vi "Read Model from JSON.vi"(8 "error in (no error)":errorcluster, 11 "JSON string":string) -> (0 "error out":errorcluster, 1 "threshold for anomaly detection":T1, 3 "model out":refnum<class "AML Analytics Model.lvclass">, 4 "custom info":cluster{"key":string, "value":string}[](array[cluster]))   [LabVIEW 2017, in "MachineLearning.lvlib"]
doc: "Converts the JSON string from a saved model file to a model reference for deployment."
uses:
  MachineLearning.lvlib
  <vilib>/addons/AML/Common/Classes/AML Analytics Model.lvclass
  <vilib>/addons/AML/Example Support/aml_All Models (enum).ctl
  <vilib>/addons/AML/Feature Manipulation/Common/Controls/aml_Feature Manipulation Model Type.ctl
  <vilib>/addons/AML/Anomaly Detection/Common/Controls/aml_Anomaly Detection Model Type.ctl
  <vilib>/addons/AML/Clustering/Common/Controls/aml_Clustering Model Type.ctl
  <vilib>/addons/AML/Classification/Common/Controls/aml_Classification Model Type.ctl
  TypeDefs/JSONpath.ctl
  TypeDefs/All Models.ctl
  <vilib>/addons/AML/Feature Manipulation/PCA/Controls/aml_PCA Properties.ctl
  <vilib>/addons/AML/Anomaly Detection/PCA T2Q/Controls/aml_PCA T2Q Properties.ctl
  <vilib>/addons/AML/Anomaly Detection/GMM-CV/Controls/aml_ GMM-CV Model Parameters.ctl
  <vilib>/addons/AML/Clustering/GMM/Controls/aml_GMM Parameter.ctl
  <vilib>/addons/AML/Anomaly Detection/GMM-CV/Controls/aml_ GMM-CV Trained Model.ctl
  <vilib>/addons/AML/Clustering/DBSCAN/Controls/aml_DBSCAN Model.ctl
  <vilib>/addons/AML/Clustering/K-Means/Controls/aml_Kmeans Model.ctl
  <vilib>/addons/AML/Clustering/GMM/Controls/aml_GMM Model.ctl
  <vilib>/addons/AML/Classification/Logistic Regression/Controls/aml_Logistic Regression Model.ctl
  <vilib>/addons/AML/Classification/Common/Classes/AML Classification.lvclass/AML Classification.ctl
  <vilib>/addons/AML/Classification/Logistic Regression/Classes/AML Logistic Regression.lvclass/AML Logistic Regression.ctl
  <vilib>/addons/AML/Common/Classes/AML Analytics Model.lvclass/AML Analytics Model.ctl
  <vilib>/addons/AML/Classification/Set Classification Model (LR).vi
  <vilib>/addons/AML/Classification/Logistic Regression/Classes/aml_Write Coefficients.vi
  <vilib>/addons/AML/Classification/Common/Classes/aml_Write Number of Classes.vi
  <vilib>/addons/AML/Classification/Common/Classes/aml_Write Label of Each Class.vi
  <vilib>/addons/AML/Common/Classes/aml_Write AML Classification Model.vi
  <vilib>/addons/AML/Classification/Common/Classes/aml_Write Model Status.vi
  <vilib>/addons/AML/Classification/Common/Classes/aml_Write Classification Model Type.vi
  <vilib>/addons/AML/Common/Classes/aml_Write Classification Model Type.vi
  <vilib>/addons/AML/Classification/Common/Classes/aml_Read Classification Model Type.vi
  <vilib>/addons/AML/Classification/Logistic Regression/Classes/AML Logistic Regression.lvclass
  C:/Program Files (x86)/National Instruments/LabVIEW 2017/vi.lib/addons/AML/Classification/Common/Classes/AML Classification.lvclass
  <vilib>/addons/AML/Classification/Logistic Regression/subVIs/aml_Check LR Model.vi
  <vilib>/addons/AML/Classification/Set Classification Model (NN).vi
  <vilib>/addons/AML/Classification/Set Classification Model (SVM).vi
  <vilib>/addons/AML/Clustering/Set Clustering Model (GMM).vi
  <vilib>/addons/AML/Clustering/Set Clustering Model (K-Means).vi
  <vilib>/addons/AML/Clustering/Set Clustering Model (DBSCAN).vi
  <vilib>/addons/AML/Anomaly Detection/Set Anomaly Detection Model (One-Class SVM).vi
  <vilib>/addons/AML/Anomaly Detection/Set Anomaly Detection Model (GMM-CV).vi
  <vilib>/addons/AML/Anomaly Detection/Set Anomaly Detection Model (PCA T2Q).vi
  <vilib>/addons/AML/Anomaly Detection/Set Anomaly Detection Model (SOM-MQE).vi
  <vilib>/addons/AML/Feature Manipulation/Set Feature Manipulation Model (KPCA).vi
  <vilib>/addons/AML/Feature Manipulation/Set Feature Manipulation Model (PCA).vi
  <vilib>/addons/AML/Feature Manipulation/Set Feature Manipulation Model (Fisher).vi
  <vilib>/addons/AML/Feature Manipulation/Set Feature Manipulation Model (Normalize).vi
  <vilib>/addons/AML/Analytics and Machine Learning.lvlib
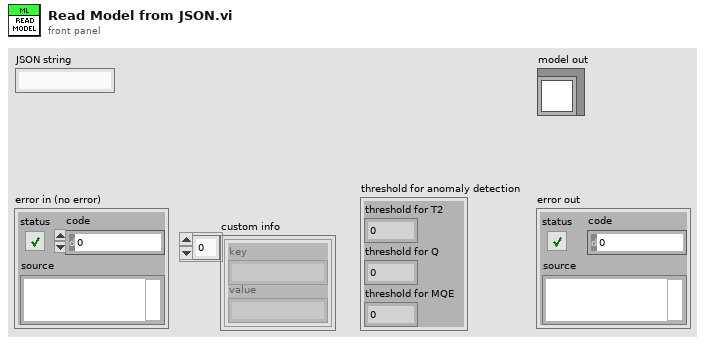
[diagram p1: front panel]
types:
  T1 = cluster{"threshold for T2":dbl, "threshold for Q":dbl, "threshold for MQE":dbl}
  T2 = typedef "All Models.ctl" = cluster{u16[], u16, u16, u16}
  T3 = typedef "MachineLearning.lvlib/JSONpath.ctl" = enum16{"Training Time", "All Models", "Feature Manipulation", "Anomaly Detection", "Clustering", "Classification", "Custom Info"}
  T4 = typedef "aml_All Models (enum).ctl" = cluster{"feature manipulation":T5[], "anomaly detection model type":T6, "clustering model type":T7, "classification model type":T8}
  T5 = typedef "Analytics and Machine Learning.lvlib/aml_Feature Manipulation Model Type.ctl" = enum16{"None", "Normalize", "Fisher", "PCA", "KPCA"}
  T6 = typedef "Analytics and Machine Learning.lvlib/aml_Anomaly Detection Model Type.ctl" = enum16{"None", "SOM-MQE", "PCA T2Q", "GMM-CV", "One-class SVM"}
  T7 = typedef "Analytics and Machine Learning.lvlib/aml_Clustering Model Type.ctl" = enum16{"None", "DBSCAN", "K-Means", "GMM"}
  T8 = typedef "Analytics and Machine Learning.lvlib/aml_Classification Model Type.ctl" = enum16{"None", "SVM", "Neural Network", "Logistic Regression", "Multi-Layer Neural Network"}
  T9 = cluster{"normalization settings":cluster{"transformation method":i32, "range settings":cluster{"max":dbl, "min":dbl}}, "mean values":dbl[], "standard deviation values":dbl[], "min values":dbl[], "max values":dbl[]}
  T10 = typedef "Analytics and Machine Learning.lvlib/aml_PCA Properties.ctl" = cluster{"mean values":dbl[], "eigenvectors":dbl[][]}
  T11 = cluster{"kernel settings":cluster{"type":i32, "degree":i32, "gamma":dbl, "coef0":dbl}, "variance":dbl[], "source data":dbl[][], "eigenvectors":dbl[][]}
  T12 = cluster{"map vectors":dbl[][], "MQE threshold":dbl, "map structure":cluster{"row":i32, "col":i32, "lattice type":i32}}
  T13 = typedef "Analytics and Machine Learning.lvlib/aml_PCA T2Q Properties.ctl" = cluster{"mean values":dbl[], "eigenvectors":dbl[][], "variance":dbl[], "threshold for T2":dbl, "threshold for Q":dbl}
  T14 = typedef "Analytics and Machine Learning.lvlib/aml_ GMM-CV Model Parameters.ctl" = cluster{"hyperparameters":T15, "baseline model":T16}
  T15 = typedef "Analytics and Machine Learning.lvlib/aml_GMM Parameter.ctl" = cluster{"auto initialization":bool, "initial mean values":dbl[][], "initial covariance values":cluster{"initial covariance matrix":dbl[][]}[], "initial weights":dbl[], "number of clusters":i32, "regulator":dbl, "tolerance":dbl, "max iteration":i32}
  T16 = typedef "Analytics and Machine Learning.lvlib/aml_ GMM-CV Trained Model.ctl" = cluster{"weights":dbl[], "covariance values":cluster{"covariance matrix":dbl[][]}[], "mean values":dbl[][]}
  T17 = cluster{"kernel settings":cluster{"type":i32, "degree":i32, "gamma":dbl, "coef0":dbl}, "number of support vectors":i32, "support vectors":dbl[][], "coeffcients of support vectors":dbl[][], "decision function constants":dbl[]}
  T18 = typedef "Analytics and Machine Learning.lvlib/aml_DBSCAN Model.ctl" = cluster{"max distance":dbl, "p":dbl, "core samples":dbl[][], "core samples labels":i32[]}
  T19 = typedef "Analytics and Machine Learning.lvlib/aml_Kmeans Model.ctl" = cluster{"centroids":dbl[][], "number of clusters":i32}
  T20 = typedef "Analytics and Machine Learning.lvlib/aml_GMM Model.ctl" = cluster{"number of clusters":i32, "mean values":dbl[][], "covariance values":cluster{"covariance matrix":dbl[][]}[], "weights":dbl[]}
  T21 = cluster{"kernel settings":cluster{"type":dbl, "degree":i32, "gamma":dbl, "coef0":dbl}, "number of classes":i32, "label of each class":i32[], "number of support vectors":i32, "support vectors":dbl[][], "coeffcients of support vectors":dbl[][], "decision function constants":dbl[], "pairwise probability":cluster{"probA":dbl[], "probB":dbl[]}, "number of support vectors for each class":i32[]}
  T22 = cluster{"number of classes":i32, "label of each class":i32[], "number of input neurons":i32, "number of hidden neurons":i32, "number of output neurons":i32, "hidden layer type":i32, "output layer type":i32, "I to H coefficients":dbl[][], "H to O coefficients":dbl[][]}
  T23 = typedef "Analytics and Machine Learning.lvlib/aml_Logistic Regression Model.ctl" = cluster{"number of classes":i32, "label of each class":i32[], "coefficients":dbl[][]}
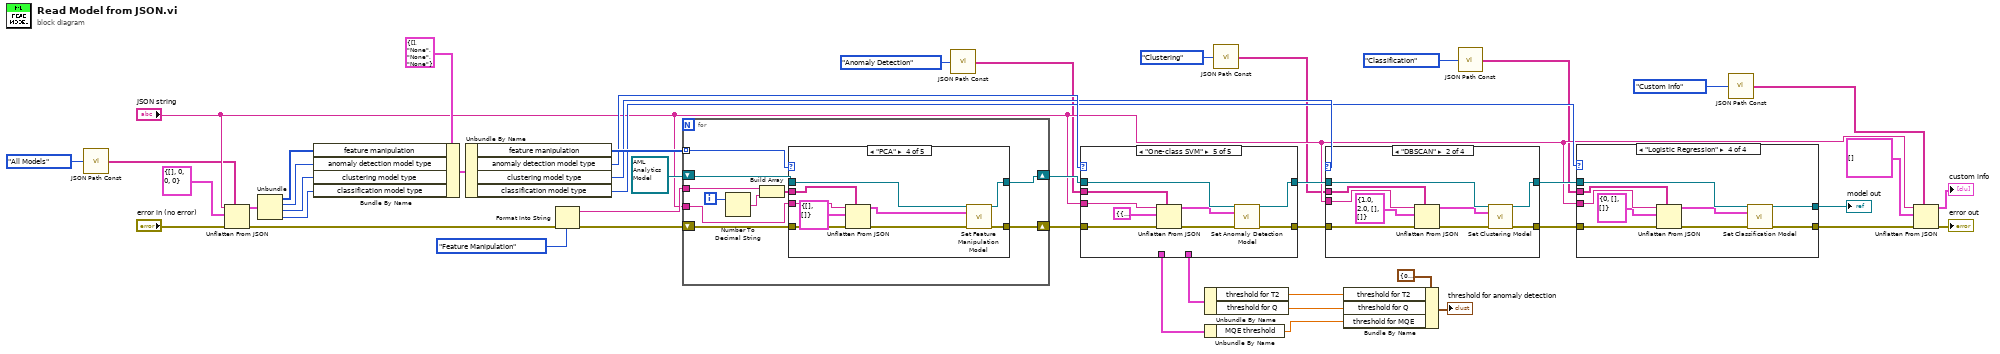
[diagram p0: block diagram]
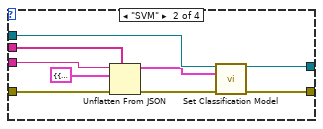
[diagram p3: hidden frame]
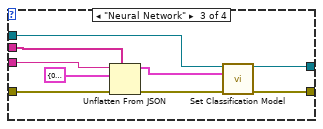
[diagram p4: hidden frame]
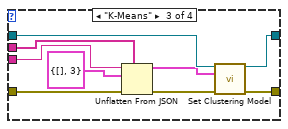
[diagram p6: hidden frame]
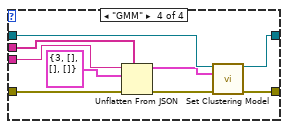
[diagram p7: hidden frame]
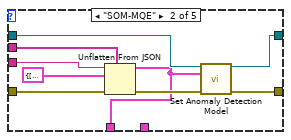
[diagram p9: hidden frame]
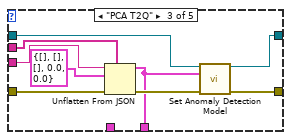
[diagram p10: hidden frame]
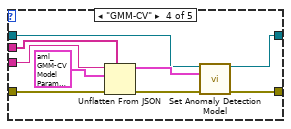
[diagram p11: hidden frame]
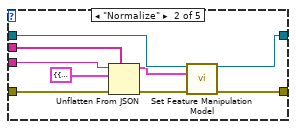
[diagram p13: hidden frame]
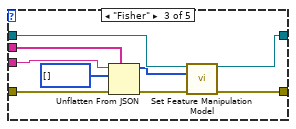
[diagram p14: hidden frame]
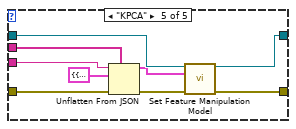
[diagram p15: hidden frame]
diagram:
  n1 = call "JSON Path Const.vi"("JSON Path"=JSONpath."All Models") -> ("resulting array"=w11:string[])
  n2 = Unflatten From JSON(path=w11, JSON string="JSON string", type and defaults=T2 {[], 0, 0, 0} ("cluster"), error in (no error)="error in (no error)") -> (value=w46:T2, error out=w26:errorcluster)  [unwired: 3 in]
  n3 = Unbundle(w46) -> (w41:u16[], w44:u16, w43:u16, w42:u16)
  n4 = Bundle By Name(cluster=T4 {"feature manipulation"=[], "anomaly detection model type"=enum."None", "clustering model type"=enum."None", "classification model type"=enum."None"}, "feature manipulation"=w41, "anomaly detection model type"=w44, "clustering model type"=w43, "classification model type"=w42) -> (w39:T4)
  n5 = Unbundle By Name(w39) -> ("feature manipulation"=w38:T5[], "anomaly detection model type"=w37:T6, "clustering model type"=w34:T7, "classification model type"=w30:T8)
  n6 = Format Into String(JSONpath."Feature Manipulation" ("JSON Path")) -> (resulting string=w28:string)  [unwired: 3 in, 1 out]
  n7 = for {
    tunnel: w38 -> [w47] mode=indexing
    tunnel: "JSON string" -> [w56]
    shift-right: [w54] -> w35
    shift-left: refnum<class "AML Analytics Model.lvclass"> refnum ("model out") -> [w55]
    shift-right: [w53] -> w36
    shift-left: w26 -> [w48]
    tunnel: w28 -> [w50]
    i -> [w52]
    n8 = Number To Decimal String(number=w52) -> (decimal integer string=w51:string)  [unwired: 1 in]
    n9 = Build Array(w50, w51) -> (w49:string[])
    n10 = case shown="\"PCA\"" w47 {
      tunnel: w56 -> [_ w67 w76 w85 w94]
      tunnel: w55 -> [w58 w66 w75 w84 w93]
      tunnel: [w58 w65 w74 w83 w92] -> w54
      tunnel: [w57 w63 w72 w81 w90] -> w53
      tunnel: w49 -> [_ w62 w71 w80 w89]
      tunnel: w48 -> [w57 w61 w70 w79 w88]
      frame "None", Default {
      }
      frame "Normalize" {
        n11 = Unflatten From JSON(path=w62, JSON string=w67, type and defaults=T9 {"normalization settings"={"transformation method"=0, "range settings"={"max"=0.0, "min"=0.0}}, "mean values"=[], "standard deviation values"=[], "min values"=[], "max values"=[]} ("normalization properties"), error in (no error)=w61) -> (value=w60:T9, error out=w64:errorcluster)  [unwired: 3 in]
        n12 = call-poly <vilib>:"Set Feature Manipulation Model.vi"("model in"=w66, "normalization model"=w60, "error in (no error)"=w64) -> ("model out"=w65:refnum<class "AML Analytics Model.lvclass">, "error out"=w63:errorcluster)  [unwired: 11 in]
      }
      frame "Fisher" {
        n13 = Unflatten From JSON(path=w71, JSON string=w76, type and defaults=i32[] [] ("Selected Feature Index"), error in (no error)=w70) -> (value=w68:i32[], error out=w73:errorcluster)  [unwired: 3 in]
        n14 = call-poly <vilib>:"Set Feature Manipulation Model.vi"("model in"=w75, "selected feature index"=w68, "error in (no error)"=w73) -> ("model out"=w74:refnum<class "AML Analytics Model.lvclass">, "error out"=w72:errorcluster)  [unwired: 11 in]
      }
      frame "PCA" {
        n15 = Unflatten From JSON(path=w80, JSON string=w85, type and defaults=T10 {"mean values"=[], "eigenvectors"=[]} ("PCA properties"), error in (no error)=w79) -> (value=w77:T10, error out=w82:errorcluster)  [unwired: 3 in]
        n16 = call-poly <vilib>:"Set Feature Manipulation Model.vi"("model in"=w84, "PCA model"=w77, "error in (no error)"=w82) -> ("model out"=w83:refnum<class "AML Analytics Model.lvclass">, "error out"=w81:errorcluster)  [unwired: 11 in]
      }
      frame "KPCA" {
        n17 = Unflatten From JSON(path=w89, JSON string=w94, type and defaults=T11 {"kernel settings"={"type"=0, "degree"=3, "gamma"=1.0, "coef0"=0.0}, "variance"=[], "source data"=[], "eigenvectors"=[]} ("KPCA properties"), error in (no error)=w88) -> (value=w86:T11, error out=w91:errorcluster)  [unwired: 3 in]
        n18 = call-poly <vilib>:"Set Feature Manipulation Model.vi"("model in"=w93, "KPCA model"=w86, "error in (no error)"=w91) -> ("model out"=w92:refnum<class "AML Analytics Model.lvclass">, "error out"=w90:errorcluster)  [unwired: 11 in]
      }
    }
  }
  n19 = call "JSON Path Const.vi"("JSON Path"=JSONpath."Anomaly Detection") -> ("resulting array"=w9:string[])
  n20 = case shown="\"One-class SVM\"" w37 {
    tunnel: w36 -> [w95 w105 w114 w123 w132]
    tunnel: w35 -> [w96 w104 w113 w121 w131]
    tunnel: [w96 w103 w112 w120 w130] -> w33
    tunnel: [w95 w101 w110 w118 w128] -> w32
    tunnel: "JSON string" -> [_ w100 w109 w117 w127]
    tunnel: w9 -> [_ w99 w108 w116 w126]
    tunnel: [_ _ w106 _ _] -> w19
    tunnel: [_ w97 _ _ _] -> w18
    frame "None", Default {
    }
    frame "SOM-MQE" {
      n21 = Unflatten From JSON(path=w99, JSON string=w100, type and defaults=T12 {"map vectors"=[], "MQE threshold"=0.0, "map structure"={"row"=0, "col"=0, "lattice type"=0}} ("SOM-MQE model"), error in (no error)=w105) -> (value=w97:T12, error out=w102:errorcluster)  [unwired: 3 in]
      n22 = call-poly <vilib>:"Set Anomaly Detection Model.vi"("model in"=w104, "SOM baseline model"=w97, "error in (no error)"=w102) -> ("model out"=w103:refnum<class "AML Analytics Model.lvclass">, "error out"=w101:errorcluster)  [unwired: 11 in]
    }
    frame "PCA T2Q" {
      n23 = Unflatten From JSON(path=w108, JSON string=w109, type and defaults=T13 {"mean values"=[], "eigenvectors"=[], "variance"=[], "threshold for T2"=0.0, "threshold for Q"=0.0} ("PCA T2Q model"), error in (no error)=w114) -> (value=w106:T13, error out=w111:errorcluster)  [unwired: 3 in]
      n24 = call-poly <vilib>:"Set Anomaly Detection Model.vi"("model in"=w113, "PCA baseline model"=w106, "error in (no error)"=w111) -> ("model out"=w112:refnum<class "AML Analytics Model.lvclass">, "error out"=w110:errorcluster)  [unwired: 11 in]
    }
    frame "GMM-CV" {
      n25 = Unflatten From JSON(path=w116, JSON string=w117, type and defaults=T14 {"hyperparameters"={"auto initialization"=TRUE, "initial mean values"=[], "initial covariance values"=[], "initial weights"=[], "number of clusters"=3, "regulator"=1e-06, "tolerance"=1e-05, "max iteration"=50}, "baseline model"={"weights"=[], "covariance values"=[], "mean values"=[]}} ("GMM-CV model parameters"), error in (no error)=w123) -> (value=w122:T14, error out=w119:errorcluster)  [unwired: 3 in]
      n26 = call-poly <vilib>:"Set Anomaly Detection Model.vi"("model in"=w121, "GMM baseline model"=w122, "error in (no error)"=w119) -> ("model out"=w120:refnum<class "AML Analytics Model.lvclass">, "error out"=w118:errorcluster)  [unwired: 11 in]
    }
    frame "One-class SVM" {
      n27 = Unflatten From JSON(path=w126, JSON string=w127, type and defaults=T17 {"kernel settings"={"type"=0, "degree"=3, "gamma"=1.0, "coef0"=0.0}, "number of support vectors"=0, "support vectors"=[], "coeffcients of support vectors"=[], "decision function constants"=[]} ("One-class SVM model"), error in (no error)=w132) -> (value=w125:T17, error out=w129:errorcluster)  [unwired: 3 in]
      n28 = call-poly <vilib>:"Set Anomaly Detection Model.vi"("model in"=w131, "one-class SVM model"=w125, "error in (no error)"=w129) -> ("model out"=w130:refnum<class "AML Analytics Model.lvclass">, "error out"=w128:errorcluster)  [unwired: 11 in]
    }
  }
  n29 = Unbundle By Name(w19) -> ("threshold for T2"=w16:dbl, "threshold for Q"=w15:dbl)
  n30 = Unbundle By Name(w18) -> ("MQE threshold"=w14:dbl)
  n31 = call "JSON Path Const.vi"("JSON Path"=JSONpath."Clustering") -> ("resulting array"=w6:string[])
  n32 = case shown="\"DBSCAN\"" w34 {
    tunnel: w32 -> [w133 w143 w152 w161]
    tunnel: w33 -> [w134 w142 w151 w160]
    tunnel: [w134 w140 w149 w158] -> w31
    tunnel: [w133 w139 w148 w157] -> w29
    tunnel: "JSON string" -> [_ w138 w147 w156]
    tunnel: w6 -> [_ w137 w146 w155]
    frame "None", Default {
    }
    frame "DBSCAN" {
      n33 = Unflatten From JSON(path=w137, JSON string=w138, type and defaults=T18 {"max distance"=1.0, "p"=2.0, "core samples"=[], "core samples labels"=[]} ("DBSCAN model"), error in (no error)=w143) -> (value=w135:T18, error out=w141:errorcluster)  [unwired: 3 in]
      n34 = call-poly <vilib>:"Set Clustering Model.vi"("model in"=w142, "DBSCAN model"=w135, "error in (no error)"=w141) -> ("model out"=w140:refnum<class "AML Analytics Model.lvclass">, "error out"=w139:errorcluster)  [unwired: 11 in]
    }
    frame "K-Means" {
      n35 = Unflatten From JSON(path=w146, JSON string=w147, type and defaults=T19 {"centroids"=[], "number of clusters"=3} ("K-Means model"), error in (no error)=w152) -> (value=w145:T19, error out=w150:errorcluster)  [unwired: 3 in]
      n36 = call-poly <vilib>:"Set Clustering Model.vi"("model in"=w151, "K-Means model"=w145, "error in (no error)"=w150) -> ("model out"=w149:refnum<class "AML Analytics Model.lvclass">, "error out"=w148:errorcluster)  [unwired: 11 in]
    }
    frame "GMM" {
      n37 = Unflatten From JSON(path=w155, JSON string=w156, type and defaults=T20 {"number of clusters"=3, "mean values"=[], "covariance values"=[], "weights"=[]} ("GMM model"), error in (no error)=w161) -> (value=w153:T20, error out=w159:errorcluster)  [unwired: 3 in]
      n38 = call-poly <vilib>:"Set Clustering Model.vi"("model in"=w160, "GMM model"=w153, "error in (no error)"=w159) -> ("model out"=w158:refnum<class "AML Analytics Model.lvclass">, "error out"=w157:errorcluster)  [unwired: 11 in]
    }
  }
  n39 = Bundle By Name(cluster=T1 {"threshold for T2"=0.0, "threshold for Q"=0.0, "threshold for MQE"=0.0} ("threshold"), "threshold for T2"=w16, "threshold for Q"=w15, "threshold for MQE"=w14) -> (→"threshold for anomaly detection":T1)
  n40 = call "JSON Path Const.vi"("JSON Path"=JSONpath."Classification") -> ("resulting array"=w4:string[])
  n41 = case shown="\"Logistic Regression\"" w30 {
    tunnel: w29 -> [w162 w172 w181 w190]
    tunnel: w31 -> [w163 w170 w179 w188]
    tunnel: [w163 w168 w176 w185] -> w20
    tunnel: "JSON string" -> [_ w171 w180 w189]
    tunnel: w4 -> [_ w167 w175 w184]
    tunnel: [w162 w166 w174 w183] -> w25
    frame "None", Default {
    }
    frame "SVM" {
      n42 = Unflatten From JSON(path=w167, JSON string=w171, type and defaults=T21 {"kernel settings"={"type"=0.0, "degree"=3, "gamma"=1.0, "coef0"=0.0}, "number of classes"=0, "label of each class"=[], "number of support vectors"=0, "support vectors"=[], "coeffcients of support vectors"=[], "decision function constants"=[], "pairwise probability"={"probA"=[], "probB"=[]}, "number of support vectors for each class"=[]} ("SVM model"), error in (no error)=w172) -> (value=w164:T21, error out=w169:errorcluster)  [unwired: 3 in]
      n43 = call-poly <vilib>:"Set Classification Model.vi"("model in"=w170, "SVM model"=w164, "error in"=w169) -> ("model out"=w168:refnum<class "AML Analytics Model.lvclass">, "error out"=w166:errorcluster)  [unwired: 11 in]
    }
    frame "Neural Network" {
      n44 = Unflatten From JSON(path=w175, JSON string=w180, type and defaults=T22 {"number of classes"=0, "label of each class"=[], "number of input neurons"=0, "number of hidden neurons"=0, "number of output neurons"=0, "hidden layer type"=0, "output layer type"=0, "I to H coefficients"=[], "H to O coefficients"=[]} ("neural network model"), error in (no error)=w181) -> (value=w178:T22, error out=w177:errorcluster)  [unwired: 3 in]
      n45 = call-poly <vilib>:"Set Classification Model.vi"("model in"=w179, "neural network model"=w178, "error in (no error)"=w177) -> ("model out"=w176:refnum<class "AML Analytics Model.lvclass">, "error out"=w174:errorcluster)  [unwired: 11 in]
    }
    frame "Logistic Regression" {
      n46 = Unflatten From JSON(path=w184, JSON string=w189, type and defaults=T23 {"number of classes"=0, "label of each class"=[], "coefficients"=[]} ("logistic regression model"), error in (no error)=w190) -> (value=w187:T23, error out=w186:errorcluster)  [unwired: 3 in]
      n47 = call-poly <vilib>:"Set Classification Model.vi"("model in"=w188, "logistic regression model"=w187, "error in (no error)"=w186) -> ("model out"=w185:refnum<class "AML Analytics Model.lvclass">, "error out"=w183:errorcluster)  [unwired: 11 in]
    }
  }
  "model out" <- w20
  n48 = call "JSON Path Const.vi"("JSON Path"=JSONpath."Custom Info") -> ("resulting array"=w2:string[])
  n49 = Unflatten From JSON(path=w2, JSON string="JSON string", type and defaults=cluster{"key":string, "value":string}[] [] ("custom info"), error in (no error)=w25) -> (value=→"custom info":cluster{"key":string, "value":string}[], error out=→"error out":errorcluster)  [unwired: 3 in]
